vi "doAction.vi"(8 "error in (no error)":errorcluster, 10 "ContextData":refnum<class "ContextData.lvclass">, 11 "Run in":refnum<class "Win.lvclass">) -> (0 "error out":errorcluster, 2 "ContextData Out":refnum<class "ContextData.lvclass">, 3 "Run out":refnum<class "Win.lvclass">)   [LabVIEW 2019, in "Win.lvclass"]
uses:
  Win.lvclass
  ContextData/ContextData.lvclass
  Player/Player.lvclass/Player.ctl
  Win.lvclass/Win.ctl
  Simon_Engine/Simon_Engine.lvclass
  Player/Player.lvclass
  Messages/simonMessages/simonMessages.lvclass
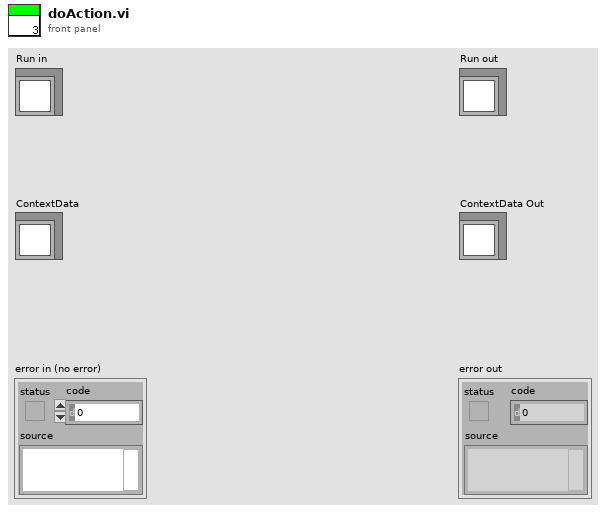
[diagram p1: front panel]
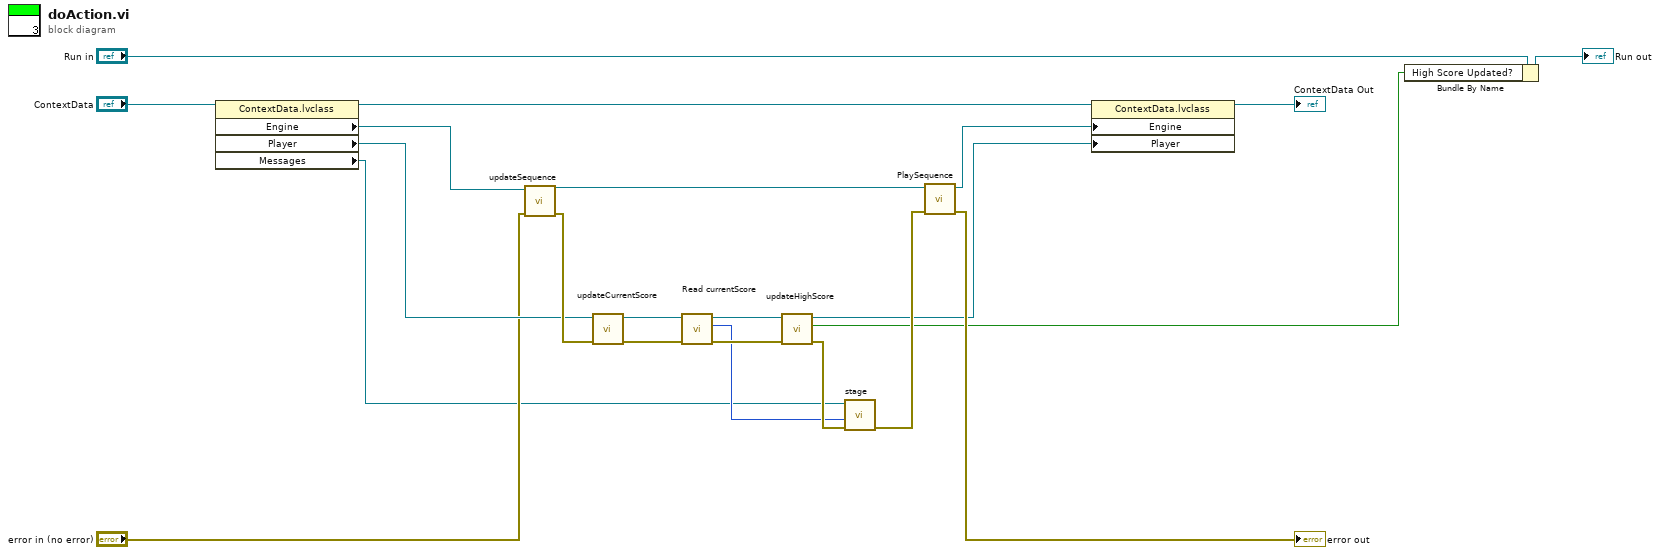
[diagram p0: block diagram]
diagram:
  n1 = property class="ContextData.lvclass"(reference="ContextData") -> (reference out=w20:refnum<class "ContextData.lvclass">, "Engine"=w8:refnum<class "Simon_Engine.lvclass">, "Player"=w7:refnum<class "Player.lvclass">, "Messages"=w3:refnum<class "simonMessages.lvclass">)  [unwired: 1 in, 1 out]
  n2 = call-dynamic "updateSequence.vi"("error in (no error)"="error in (no error)", "Simon_Engine in"=w8) -> ("error out"=w15:errorcluster, "Simon_Engine out"=w18:refnum<class "Simon_Engine.lvclass">)  [unwired: 8 in]
  n3 = call "updateCurrentScore.vi"("error in (no error)"=w15, "Player in"=w7) -> ("error out"=w14:errorcluster, "Player out"=w16:refnum<class "Player.lvclass">)  [unwired: 8 in]
  n4 = call "Read currentScore.vi"("error in (no error)"=w14, "Player in"=w16) -> ("error out"=w13:errorcluster, "currentScore"=w10:u64, "Player out"=w17:refnum<class "Player.lvclass">)  [unwired: 7 in]
  n5 = call "updateHighScore.vi"("error in (no error)"=w13, "Player in"=w17) -> ("error out"=w12:errorcluster, "High Score Updated?"=w1:bool, "Player out"=w4:refnum<class "Player.lvclass">)  [unwired: 7 in]
  n6 = call "stage.vi"("error in (no error)"=w12, "stage number"=w10, "simonMessages in"=w3) -> ("error out"=w11:errorcluster)  [unwired: 7 in, 1 out]
  n7 = call-dynamic "PlaySequence.vi"("error in (no error)"=w11, "Simon_Engine in"=w18) -> ("error out"=→"error out":errorcluster, "Simon_Engine out"=w9:refnum<class "Simon_Engine.lvclass">)  [unwired: 8 in]
  n8 = property class="ContextData.lvclass"(reference=w20, "Engine"=w9, "Player"=w4) -> (reference out=→"ContextData Out":refnum<class "ContextData.lvclass">)  [unwired: 1 in, 1 out]
  n9 = Bundle By Name(cluster="Run in", "High Score Updated?"=w1) -> (→"Run out":refnum<class "Win.lvclass">)
